vi "Write daemon status.vi"(8 "error in (no error)":errorcluster, 10 "daemon status":T1, 11 "WebSocket Server in":refnum<class "WebSocket Server.lvclass">) -> (0 "error out":errorcluster, 3 "WebSocket Server out":refnum<class "WebSocket Server.lvclass">)   [LabVIEW 2021, in "WebSockets.lvlib" / "WebSocket Server.lvclass"]
uses:
  WebSocket Server.lvclass
  daemon status.ctl
  WebSocket Server.lvclass/WebSocket Server.ctl
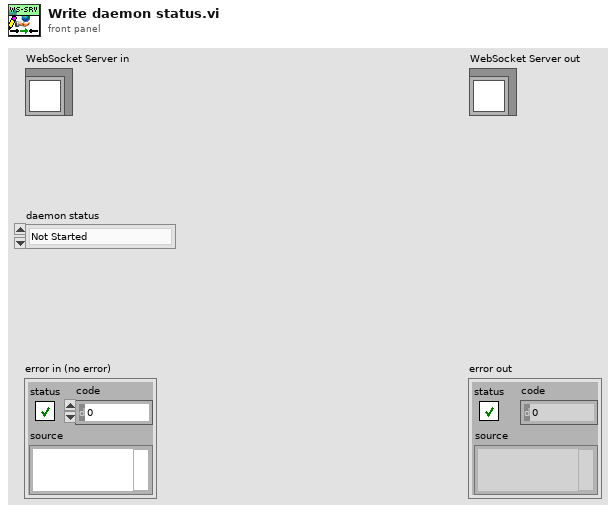
[diagram p1: front panel]
types:
  T1 = typedef "WebSockets.lvlib/WebSocket Server.lvclass/daemon status.ctl" = enum16{"Not Started", "Running", "Error", "Stopped"}
  T2 = typedef "WebSockets.lvlib/WebSocket Server.lvclass/daemon status cluster.ctl" = cluster{"error":errorcluster, "status":T1}
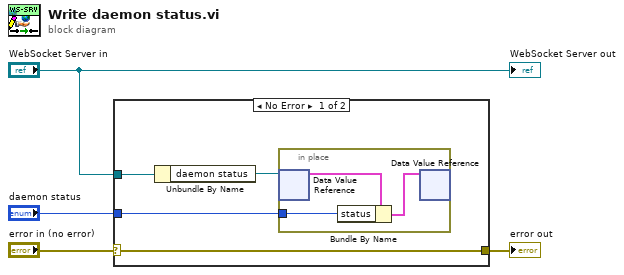
[diagram p0: block diagram]
diagram:
  n1 = case shown="No Error" "error in (no error)" {
    selector: "error in (no error)" -> [w8 w12]
    tunnel: [w8 w12] -> w3
    tunnel: "WebSocket Server in" -> [w6 _]
    tunnel: "daemon status" -> [w5 _]
    frame No Error {
      n2 = Unbundle By Name(w6) -> ("daemon status"=w7:refnum<data-value>)
      n3 = in-place {
        in-place-border: w5 -> [w9]
        n4 = in-place-dvr #1(w7) -> (w11:T2)  [unwired: 1 out]
        n5 = Bundle By Name(cluster=w11, "status"=w9) -> (w10:T2)
        n6 = in-place-dvr #1(w10) -> ()  [unwired: 2 out]
      }
    }
    frame Error {
    }
  }
  "error out" <- w3
  "WebSocket Server out" <- "WebSocket Server in"
